vi "LogToSyslog.vi"(5 "call chain level (1)":i32=1, 7 "severity (informational)":i32(ring)=2 items=["Error", "Warning", "Informational"], 10 "error in (no error)":errorcluster, 11 "message":string) -> (2 "error out":errorcluster, 3 "Syslog Message":string)   [LabVIEW 2020, in "VsDebugLibrary.lvlib"]
uses:
  VsDebugLibrary.lvlib
  <vilib>/Utility/SystemLogging/NI_SystemLogging.lvlib
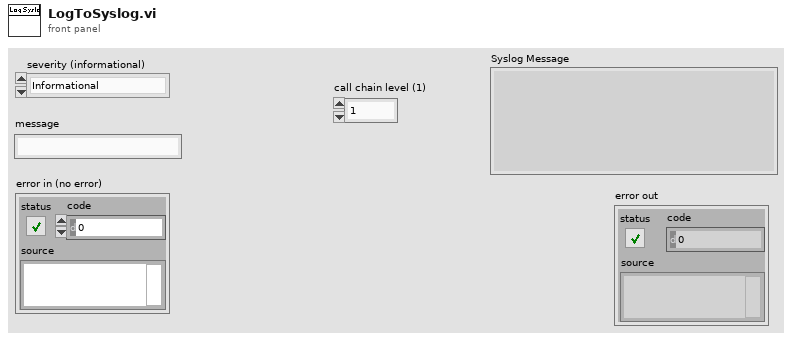
[diagram p1: front panel]
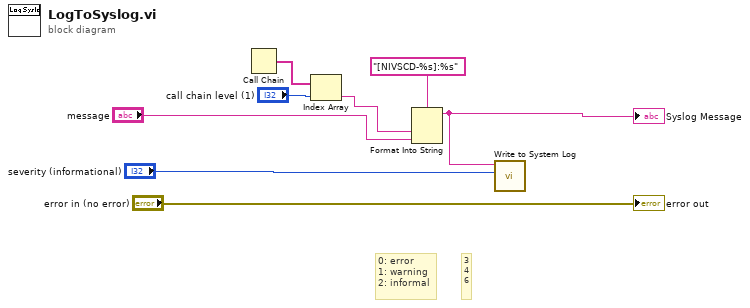
[diagram p0: block diagram]
diagram:
  # "3\n4\n6"
  # "0: error\n1: warning\n2: informal"
  n1 = Call Chain() -> (call chain=w5:string[])
  n2 = Index Array(array=w5, index="call chain level (1)") -> (element=w2:string)
  n3 = Format Into String(format string="[NIVSCD-%s]:%s", w2, "message") -> (resulting string=w6:string)  [unwired: 2 in, 1 out]
  "Syslog Message" <- w6
  n4 = call <vilib>:"Write to System Log.vi"("severity"="severity (informational)", "message"=w6) -> ()  [unwired: 9 in, 1 out]
  "error out" <- "error in (no error)"
